vi "Initialize.vi"(9 "State Variables in":T1, 10 "Item.Data":T8, 11 "NIVS.Gateway IP Address":string) -> (0 "error out":errorcluster, 3 "State Variables out":T1)   [LabVIEW 2013, in "Instrument Workspace Objects.lvlib"]
uses:
  Instrument Workspace Objects.lvlib
  Types/State Variables.ctl
  <vilib>/NI Veristand/Display Template Support/Display Template Support.llb/enum_Display Template Handler Minimal To Workspace.ctl
  <vilib>/NI Veristand/Display Template Support/Display Template Support.llb/enum_Display Template Handler Minimal To Widget Msg.ctl
  NationalInstruments.VeriStand.SystemStorage
  <vilib>/NI Veristand/Execution/Workspace/WorkspaceAPI.ctl
  NationalInstruments.VeriStand.ClientAPI
  <userlib>/STM/TCP/stm_TCP Connection Info.ctl
  <userlib>/STM/_SubVIs/stm_MetaDataElement.ctl
  Types/CD Saved State.ctl
  <vilib>/NI Veristand/Execution/Workspace/SystemStateEventRef.ctl
  <vilib>/NI Veristand/Execution/Workspace/SystemStateRegEventRef.ctl
  <vilib>/NI Veristand/Display Template Support/Display Template Support.llb/cluster_Screen Item Settings.ctl
  <vilib>/NI Veristand/Display Template Support/Display Template Support.llb/cluster_Graph Scale Settings.ctl
  <vilib>/NI Veristand/Display Template Support/Display Template Support.llb/cluster_Graph Plot Settings.ctl
  <vilib>/NI Veristand/Execution/Workspace/NI_VS Workspace ExecutionAPI.lvlib
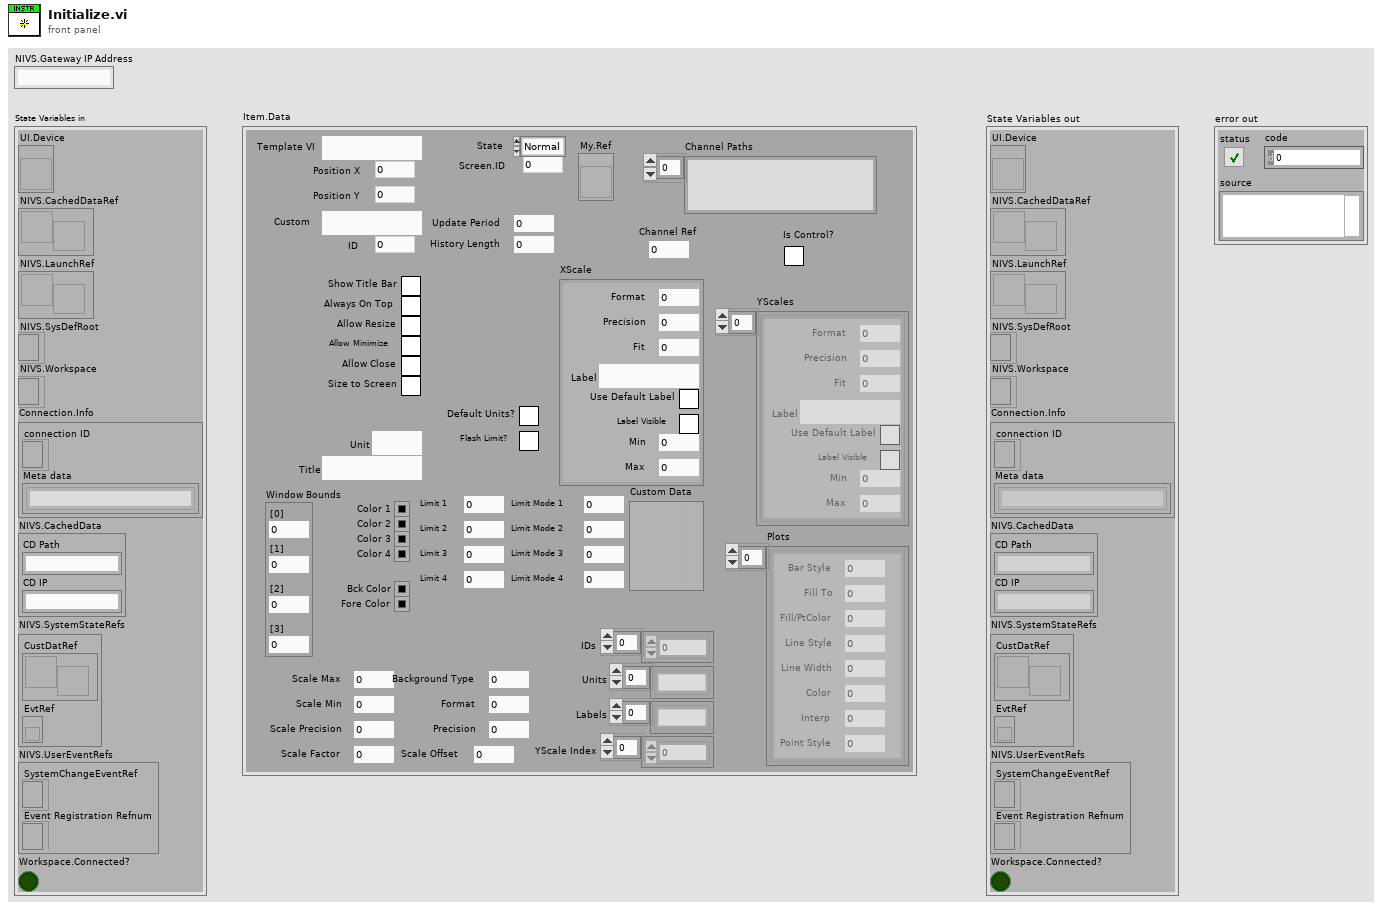
[diagram p1: front panel]
types:
  T1 = typedef "Instrument Workspace Objects.lvlib/State Variables.ctl" = cluster{"UI.Device":refnum<vi>, "NIVS.CachedDataRef":refnum<user-event>, "NIVS.LaunchRef":refnum<user-event>, "NIVS.SysDefRoot":refnum<k24>, "NIVS.Workspace":T2, "Connection.Info":T3, "NIVS.CachedData":T5, "NIVS.SystemStateRefs":T6, "NIVS.UserEventRefs":cluster{"SystemChangeEventRef":T7, "Event Registration Refnum":refnum<event-registration>}, "Workspace.Connected?":bool}
  T2 = typedef "NI_VS Workspace ExecutionAPI.lvlib/WorkspaceAPI.ctl" = refnum<k24>
  T3 = typedef "stm_TCP Connection Info.ctl" = cluster{"connection ID":refnum<k5>, "Meta data":T4[]}
  T4 = typedef "stm_MetaDataElement.ctl" = string
  T5 = typedef "Instrument Workspace Objects.lvlib/CD Saved State.ctl" = cluster{"CD Path":string, "CD IP":string}
  T6 = typedef "NI_VS Workspace ExecutionAPI.lvlib/SystemStateEventRef.ctl" = cluster{"CustDatRef":refnum<user-event>, "EvtRef":refnum<k27>}
  T7 = typedef "NI_VS Workspace ExecutionAPI.lvlib/SystemStateRegEventRef.ctl" = refnum<event-registration>
  T8 = typedef "cluster_Screen Item Settings.ctl" = cluster{"Template VI":string, "Position X":i32, "Position Y":i32, "Custom":string, "Show Title Bar":bool, "ID":i32, "Always On Top":bool, "Allow Resize":bool, "Allow Minimize":bool, "Allow Close":bool, "Size to Screen":bool, "Screen.ID":i32, "State":enum16{"Normal", "New"}, "Title":string, "Window Bounds":cluster{"[0]":i16, "[1]":i16, "[2]":i16, "[3]":i16}, "Channel Ref":u64, "Unit":string, "Default Units?":bool, "Flash Limit?":bool, "Color 1":u32, "Color 2":u32, "Color 3":u32, "Color 4":u32, "Bck Color":u32, "Fore Color":u32, "Limit 1":dbl, "Limit 2":dbl, "Limit 3":dbl, "Limit 4":dbl, "Limit Mode 1":i32, "Limit Mode 2":i32, "Limit Mode 3":i32, "Limit Mode 4":i32, "Scale Precision":i32, "Scale Min":dbl, "Scale Max":dbl, "Format":i32, "Precision":i32, "Background Type":i32, "IDs":i32[], "Units":string[], "Labels":string[], "Scale Factor":dbl, "Scale Offset":dbl, "YScale Index":u32[], "XScale":T9, "YScales":T9[], "Plots":T10[], "Update Period":dbl, "History Length":dbl, "My.Ref":refnum<vi>, "Is Control?":bool, "Channel Paths":string[], "Custom Data":variant}
  T9 = typedef "cluster_Graph Scale Settings.ctl" = cluster{"Format":u8, "Precision":u8, "Fit":u8, "Label":string, "Use Default Label":bool, "Label Visible":bool, "Min":dbl, "Max":dbl}
  T10 = typedef "cluster_Graph Plot Settings.ctl" = cluster{"Bar Style":u8, "Fill To":i16, "Fill/PtColor":u32, "Line Style":u8, "Line Width":u8, "Color":u32, "Interp":u8, "Point Style":u8}
  T11 = cluster{"SystemChangeEventRef":T7, "Event Registration Refnum":refnum<event-registration>}
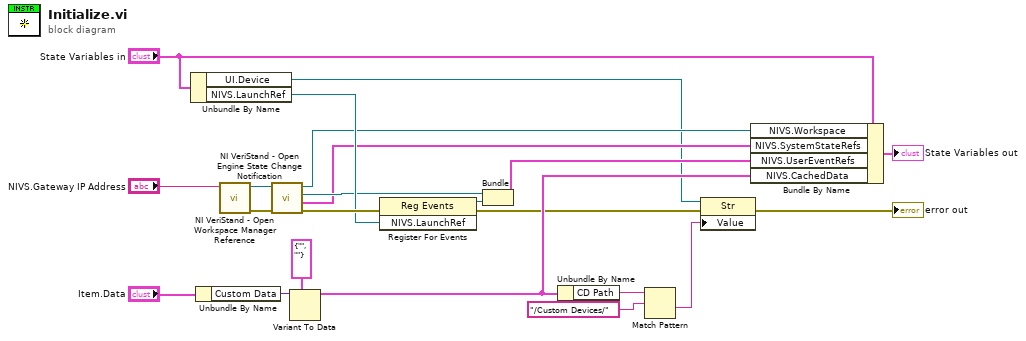
[diagram p0: block diagram]
diagram:
  n1 = Unbundle By Name("State Variables in") -> ("UI.Device"=w3:refnum<vi>, "NIVS.LaunchRef"=w14:refnum<user-event>)
  n2 = Unbundle By Name("Item.Data") -> ("Custom Data"=w18:variant)
  n3 = call <vilib>:"NI VeriStand - Open Workspace Manager Reference.vi"("Gateway IP Address (\"\": localhost)"="NIVS.Gateway IP Address") -> ("error out"=w20:errorcluster, "WorkspaceManager"=w21:T2)  [unwired: 9 in]
  n4 = call <vilib>:"NI VeriStand - Open Engine State Change Notification.vi"("error in (no error)"=w20, "WorkspaceManager in"=w21) -> ("error out"=w17:errorcluster, "SystemStateRefs"=w10:T6, "SystemChangeEventRef"=w13:T7, "WorkspaceManager out"=w11:T2)  [unwired: 6 in]
  n5 = Variant To Data(type=T5 {"CD Path"="", "CD IP"=""}, Variant=w18) -> (data=w6:T5)  [unwired: 1 in, 1 out]
  n6 = register-events(error in=w17, w14) -> (reference out=w22:refnum<event-registration>, error out=w5:errorcluster)  [unwired: 1 in]
  n7 = Bundle("SystemChangeEventRef"=w13, "Event Registration Refnum"=w22) -> (w9:T11)  [unwired: 1 in]
  n8 = Unbundle By Name(w6) -> ("CD Path"=w1:string)
  n9 = Match Pattern(string=w1, regular expression="/Custom Devices/") -> (after substring=w2:string)  [unwired: 1 in, 3 out]
  n10 = property class="Str"(reference=w3, error in=w5, "Value"=w2) -> (error out=→"error out":errorcluster)  [unwired: 1 out]
  n11 = Bundle By Name(cluster="State Variables in", "NIVS.Workspace"=w11, "NIVS.SystemStateRefs"=w10, "NIVS.UserEventRefs"=w9, "NIVS.CachedData"=w6) -> (→"State Variables out":T1)
